vi "pharosTriggersDoubleTrainGenerate.vi"(1 "off at the end":bool=TRUE, 2 "time btwn trains (s)":dbl, 3 "n trains":i32) -> (0 "triggers":u8[](array[numeric]))   [LabVIEW 2017]
uses:
  globalUtilities.vi
  globalDevices.vi
panel:
  out "Boolean array":bool[][](array[boolean])
  out "x-y":dbl
  out "size(s)":i32
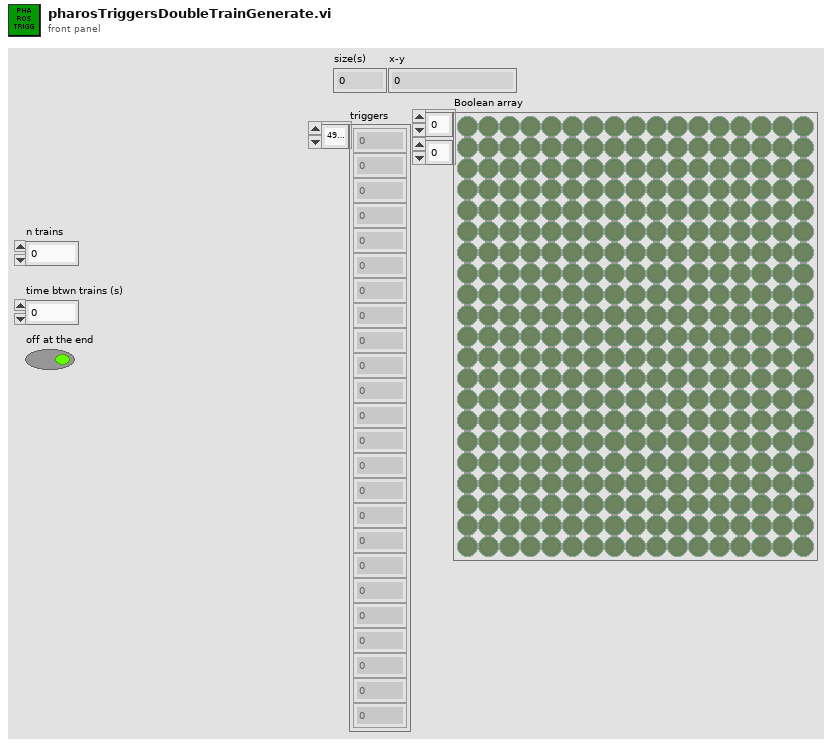
[diagram p1: front panel]
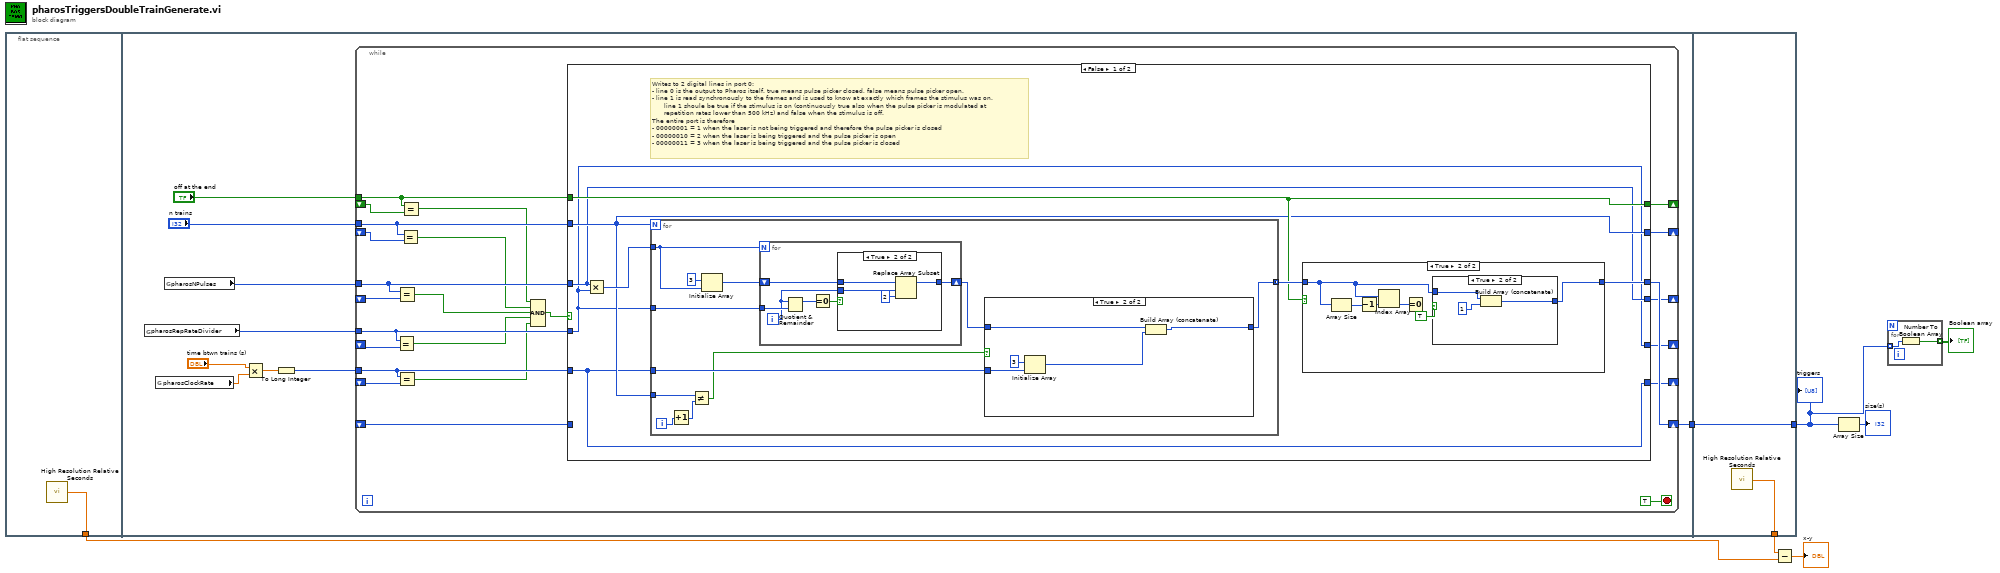
[diagram p0: block diagram]
diagram:
  n1 = flat-sequence {
    tunnel: [w8] -> w4
    tunnel: [w14] -> w6
    tunnel: [w96] -> w2
    tunnel: w6 -> [w96]
    tunnel: [w95] -> w5
    frame #0 {
      n2 = call <vilib>:"High Resolution Relative Seconds.vi"() -> ("relative seconds"=w8:dbl)
    }
    frame #1 {
      n3 = global read "globalUtilities.vi" "pharosRepRateDivider"() -> (w17:i32)
      n4 = global read "globalDevices.vi" "pharosClockRate"() -> (w11:dbl)
      n5 = global read "globalUtilities.vi" "pharosNPulses"() -> (w16:i32)
      n6 = Multiply(x="time btwn trains (s)", y=w11) -> (x*y=w10:dbl)
      n7 = To Long Integer(number=w10) -> (32bit integer=w9:i32)
      n8 = while {
        tunnel: w17 -> [w29]
        tunnel: w16 -> [w31]
        tunnel: "off at the end" -> [w35]
        tunnel: "n trains" -> [w33]
        tunnel: w9 -> [w27]
        shift-right: [w40] -> _
        shift-left: _ -> [w34]
        shift-right: [w39] -> _
        shift-left: _ -> [w32]
        shift-right: [w38] -> _
        shift-left: _ -> [w30]
        shift-right: [w37] -> _
        shift-left: _ -> [w28]
        shift-right: [w36] -> _
        shift-left: _ -> [w26]
        shift-right: [w41] -> w14
        shift-left: _ -> [w19]
        stop <- TRUE stop-if-true
        n9 = Equal?(x=w29, y=w28) -> (x = y?=w22:bool)
        n10 = Equal?(x=w31, y=w30) -> (x = y?=w23:bool)
        n11 = Equal?(x=w27, y=w26) -> (x = y?=w21:bool)
        n12 = Equal?(x=w33, y=w32) -> (x = y?=w24:bool)
        n13 = Equal?(x=w35, y=w34) -> (x = y?=w25:bool)
        n14 = Compound Arithmetic op=AND(w25, w24, w23, w22, w21) -> (w20:bool)
        n15 = case shown="False" w20 {
          tunnel: w29 -> [w43 w91]
          tunnel: w31 -> [w44 w92]
          tunnel: w35 -> [w46 w94]
          tunnel: [w47 w89] -> w41
          tunnel: w33 -> [w45 w93]
          tunnel: w27 -> [w42 w90]
          tunnel: [w46 w94] -> w40
          tunnel: [w45 w93] -> w39
          tunnel: [w44 w92] -> w38
          tunnel: [w43 w91] -> w37
          tunnel: [w42 w90] -> w36
          tunnel: w19 -> [_ w89]
          frame False {
            # "Writes to 2 digital lines in port 0:\n- line 0 is the output to Pharos itself. true means pulse picker closed, false means pulse picker open.\n- line 1 is read synchronously to the frames and is used to know at exactly which frames the stimulus was on.\n      line 1 shoule be true if the stimulus is on (continuously true also when the pulse picker is modulated at\n      repetition rates lower than 500 kHz) and false when the stimulus is off.\nThe entire port is therefore\n- 00000001 = 1 when the laser is not being triggered and therefore the pulse picker is closed\n- 00000010 = 2 when the laser is being triggered and the pulse picker is open\n- 00000011 = 3 when the laser is being triggered and the pulse picker is closed"
            n16 = Multiply(x=w44, y=w43) -> (x*y=w49:i32)
            n17 = for {
              N: w45 -> [_]
              tunnel: w43 -> [w58]
              tunnel: w49 -> [w57]
              tunnel: [w50] -> w48 mode=concatenating
              tunnel: w45 -> [w54]
              tunnel: w42 -> [w53]
              i -> [w56]
              n18 = Increment(x=w56) -> (x+1=w55:i32)
              n19 = Not Equal?(x=w54, y=w55) -> (x != y?=w52:bool)
              n20 = Initialize Array(u8 3 ("element"), w57) -> (w59:u8[])
              n21 = for {
                N: w57 -> [_]
                tunnel: w58 -> [w71]
                shift-right: [w67] -> w51
                shift-left: w59 -> [w72]
                i -> [w68]
                n22 = Quotient & Remainder(x=w68, y=w71) -> (x-y*floor(x/y)=w70:i32)  [unwired: 1 out]
                n23 = Equal To 0?(x=w70) -> (x = 0?=w69:bool)
                n24 = case shown="True" w69 {
                  tunnel: w72 -> [w73 w77]
                  tunnel: w68 -> [_ w76]
                  tunnel: [w73 w74] -> w67
                  frame False {
                  }
                  frame True {
                    n25 = Replace Array Subset(array=w77, new element=u8 2 ("new element/subarray"), index=w76) -> (w74:u8[])
                  }
                }
              }
              n26 = case shown="True" w52 {
                tunnel: w53 -> [_ w65]
                tunnel: w51 -> [w61 w64]
                tunnel: [w61 w62] -> w50
                frame False {
                }
                frame True {
                  n27 = Initialize Array(u8 3 ("element"), w65) -> (w63:u8[])
                  n28 = Build Array (concatenate)(w64, w63) -> (w62:u8[])
                }
              }
            }
            n29 = case shown="True" w46 {
              tunnel: w48 -> [w78 w82]
              tunnel: [w78 w81] -> w47
              frame False {
              }
              frame True {
                n30 = Array Size(array=w82) -> (size(s)=w83:i32)
                n31 = Decrement(x=w83) -> (x-1=w80:i32)
                n32 = Index Array(array=w82, index=w80) -> (element=w84:u8)
                n33 = Equal To 0?(x=w84) -> ()  [unwired: 1 out]
                n34 = case shown="True" TRUE {
                  tunnel: w82 -> [w85 w88]
                  tunnel: [w85 w86] -> w81
                  frame False {
                  }
                  frame True {
                    n35 = Build Array (concatenate)(w88, u8 1) -> (w86:u8[])
                  }
                }
              }
            }
          }
          frame True {
          }
        }
      }
    }
    frame #2 {
      n36 = call <vilib>:"High Resolution Relative Seconds.vi"() -> ("relative seconds"=w95:dbl)
    }
  }
  n37 = Subtract(x=w5, y=w4) -> (x-y=→"x-y":dbl)
  n38 = Array Size(array=w2) -> (size(s)=→"size(s)":i32)
  n39 = for {
    tunnel: w2 -> [w98] mode=indexing
    tunnel: [w97] -> w1 mode=indexing
    n40 = Number To Boolean Array(number=w98) -> (Boolean array=w97:bool[])
  }
  "Boolean array" <- w1
  "triggers" <- w2
